vi "ValidateLumberjackConfigDTO.vi"(8 "error in (no error)":errorcluster, 11 "BaselineDTO":T1={"schemaVersion"="", "globalThreshold"="INFO", "defaultFileAppender"={"common"={"id"="", "threshold"="INFO", "filter"={"mode"="mirror", "levelMin"="INFO", "levelMax"="INFO", "tagPrefix"=""}, "queueBound"=0, "dropPolicy"="dropOldest", "useUTC"=FALSE}, "file"={"rootFolder"="", "maxFileSize"=0, "maxFileCount"=0, "baseName"="", "extension"="", "delimiter"="", "calendarFolderTree"=FALSE}}}) -> (0 "error out":errorcluster, 3 "MergedDTO":T1={"schemaVersion"="", "globalThreshold"="INFO", "defaultFileAppender"={"common"={"id"="", "threshold"="INFO", "filter"={"mode"="mirror", "levelMin"="INFO", "levelMax"="INFO", "tagPrefix"=""}, "queueBound"=0, "dropPolicy"="dropOldest", "useUTC"=FALSE}, "file"={"rootFolder"="", "maxFileSize"=0, "maxFileCount"=0, "baseName"="", "extension"="", "delimiter"="", "calendarFolderTree"=FALSE}}})   [LabVIEW 2026, in "Lumberjack.lvlib"]
doc: "Pure DTO validation. Fail-fast checks on a merged LumberjackConfigDTO, returning a descriptive error on the first invalid field: schema version, enum-name membership, file size, and filename safety of baseName and extension (SRS-LMBR-048, codes 5020-5039). Passes the DTO through on success. No I/O.\n\nMerged DTO -> descriptive error on first invalid field (else passthrough)."
uses:
  Lumberjack.lvlib
  <vilib>/Utility/Data Type/NI_Data Type.lvlib
  TypeDefs/ConfigDTO/FilterDTO.ctl
  TypeDefs/ConfigDTO/AppenderConfigDTO.ctl
  TypeDefs/ConfigDTO/FileAppenderConfigDTO.ctl
  TypeDefs/ConfigDTO/FileConfigDTO.ctl
  TypeDefs/ConfigDTO/LumberjackConfigDTO.ctl
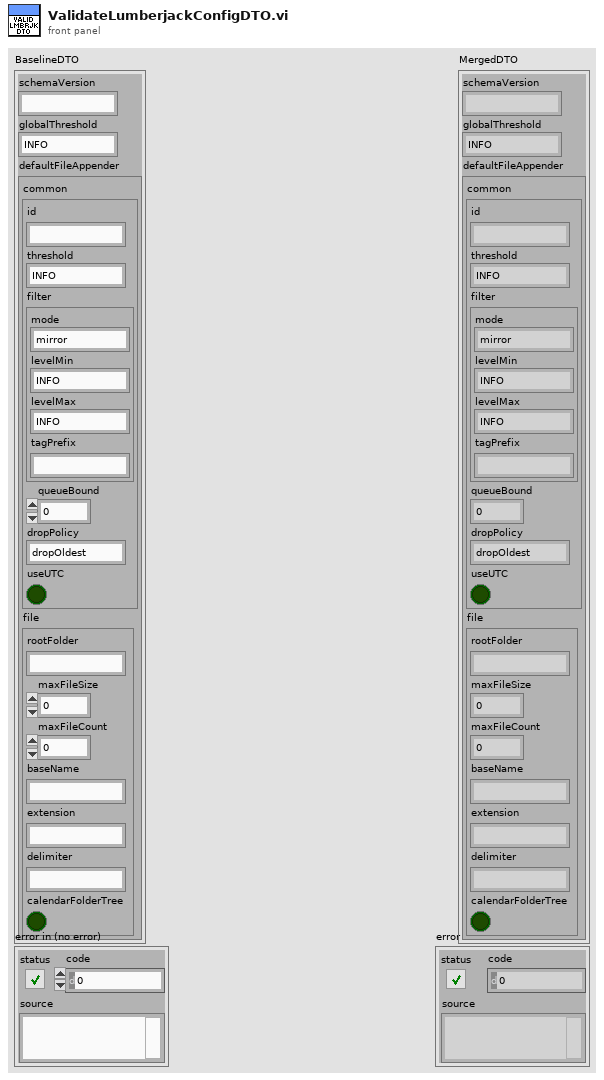
[diagram p1: front panel]
types:
  T1 = typedef "Lumberjack.lvlib/LumberjackConfigDTO.ctl" = cluster{"schemaVersion":string, "globalThreshold":string, "defaultFileAppender":T2}
  T2 = typedef "Lumberjack.lvlib/FileAppenderConfigDTO.ctl" = cluster{"common":T3, "file":T5}
  T3 = typedef "Lumberjack.lvlib/AppenderConfigDTO.ctl" = cluster{"id":string, "threshold":string, "filter":T4, "queueBound":i32, "dropPolicy":string, "useUTC":bool}
  T4 = typedef "Lumberjack.lvlib/FilterDTO.ctl" = cluster{"mode":string, "levelMin":string, "levelMax":string, "tagPrefix":string}
  T5 = typedef "Lumberjack.lvlib/FileConfigDTO.ctl" = cluster{"rootFolder":string, "maxFileSize":i64, "maxFileCount":i32, "baseName":string, "extension":string, "delimiter":string, "calendarFolderTree":bool}
  T6 = typedef "NI_Data Type.lvlib/Data Type.ctl" = enum8{"Invalid Type", "Void", "I8", "I16", "I32", "I64", "U8", "U16", "U32", "U64", "Single Float", "Double Float", "Extended Float", "Single Complex", "Double Complex", "Extended Complex", "Enum U8", "Enum U16", "Enum U32", "Enum U64", "Single Float With Unit", "Double Float With Unit", "Extended Float With Unit", "Single Complex with Unit", "Double Complex with Unit", "Extended Complex with Unit", "Boolean", "String", "Path", "Picture", "Tag", "Array", "Cluster", "Variant", "LV Variant", "Waveform", "Timestamp", "Digital Waveform", "Digital Data", "ExpressData", "Refnum", "External Data", "VI", "Poly VI", "LabVIEW Class Instance", "Fixed Point", "Set Collection", "Map Collection"}
  T7 = typedef "NI_Data Type.lvlib/Type Definition Info.ctl" = cluster{"Name":string, "Timestamp":u32}
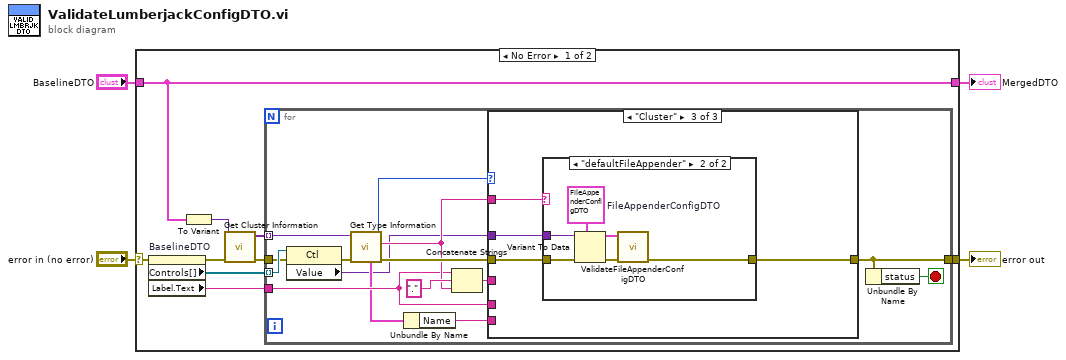
[diagram p0: block diagram]
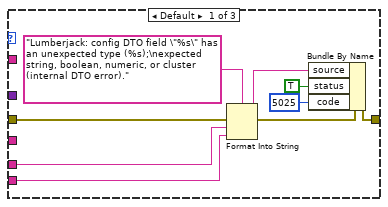
[diagram p2: hidden frame]
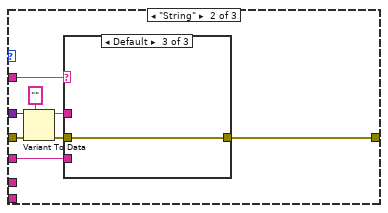
[diagram p3: hidden frame]
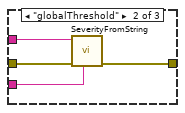
[diagram p5: hidden frame]
diagram:
  n1 = case shown="No Error" "error in (no error)" {
    selector: "error in (no error)" -> [w7 w63]
    tunnel: "BaselineDTO" -> [w5 w64]
    tunnel: [w5 w64] -> w2
    tunnel: [w6 w63] -> w1
    frame No Error {
      n2 = property on="BaselineDTO" class="Clust (strict)"(error in=w7) -> (error out=w11:errorcluster, "Controls[]"=w8:refnum<vi>[], "Label.Text"=w9:string)  [unwired: 1 in, 1 out]
      n3 = To Variant(anything=w5) -> (Variant=w10:variant)
      n4 = call <vilib>:"Get Cluster Information.vi"("error in (no error)"=w11, "variant"=w10) -> ("error out"=w12:errorcluster, "cluster elements"=w13:variant[])  [unwired: 8 in]
      n5 = for {
        tunnel: w13 -> [w23] mode=indexing
        tunnel: w12 -> [w16]
        tunnel: w9 -> [w22]
        tunnel: [w19] -> w6
        tunnel: w8 -> [w17] mode=indexing
        stop <- w18 stop-if-true
        n6 = property class="Ctl"(reference=w17, error in=w16) -> (error out=w14:errorcluster, "Value"=w15:variant)  [unwired: 1 out]
        n7 = call <vilib>:"Get Type Information.vi"("error in (no error)"=w14, "variant"=w23) -> ("error out"=w27:errorcluster, "name"=w24:string, "type"=w25:T6, "type definition info"=w21:T7)  [unwired: 5 in, 1 out]
        n8 = Unbundle By Name(w21) -> ("Name"=w20:string)
        n9 = Concatenate Strings(w22, "." ("string"), w24) -> (w26:string)
        n10 = case shown="\"Cluster\"" w25 {
          tunnel: w27 -> [w33 w43 w55]
          tunnel: w26 -> [_ w45 _]
          tunnel: w24 -> [_ w44 w53]
          tunnel: w15 -> [_ w41 w54]
          tunnel: w22 -> [w34 _ _]
          tunnel: [w30 w38 w52] -> w19
          tunnel: w20 -> [w31 _ _]
          frame Default {
            n11 = Format Into String(format string="Lumberjack: config DTO field \"%s\" has an unexpected type (%s);\nexpected string, boolean, numeric, or cluster (internal DTO error)." ("source"), error in=w33, w34, w31) -> (resulting string=w29:string, error out=w32:errorcluster)  [unwired: 1 in]
            n12 = Bundle By Name(cluster=w32, "source"=w29, "status"=TRUE, "code"=5025) -> (w30:errorcluster)
          }
          frame "String" {
            n13 = Variant To Data(error in=w43, type="", Variant=w41) -> (data=w39:string, error out=w42:errorcluster)
            n14 = case shown="Default" w44 {
              tunnel: w42 -> [w46 w50 w51]
              tunnel: w45 -> [_ w48 _]
              tunnel: w39 -> [_ w47 _]
              tunnel: [w46 w49 w51] -> w38
              frame "schemaVersion" {
              }
              frame "globalThreshold" {
                n15 = call "SeverityFromString.vi"("Context"=w48, "error in (no error)"=w50, "SeverityString"=w47) -> ("error out"=w49:errorcluster)  [unwired: 7 in, 1 out]
              }
              frame Default {
              }
            }
          }
          frame "Cluster" {
            n16 = case shown="\"defaultFileAppender\"" w53 {
              tunnel: w55 -> [w56 w62]
              tunnel: w54 -> [_ w61]
              tunnel: [w56 w58] -> w52
              frame Default {
              }
              frame "defaultFileAppender" {
                w57 = T2 {"common"={"id"="", "threshold"="INFO", "filter"={"mode"="Mirror", "levelMin"="INFO", "levelMax"="INFO", "tagPrefix"=""}, "queueBound"=0, "dropPolicy"="DropOldest", "useUTC"=FALSE}, "file"={"rootFolder"="", "maxFileSize"=0, "maxFileCount"=0, "baseName"="", "extension"="", "delimiter"="", "calendarFolderTree"=FALSE}}  # FileAppenderConfigDTO
                n17 = Variant To Data(error in=w62, type=w57, Variant=w61) -> (data=w59:T2, error out=w60:errorcluster)
                n18 = call "ValidateFileAppenderConfigDTO.vi"("error in (no error)"=w60, "FileAppenderConfigDTOin"=w59) -> ("error out"=w58:errorcluster)  [unwired: 8 in, 1 out]
              }
            }
          }
        }
        n19 = Unbundle By Name(w19) -> ("status"=w18:bool)
      }
    }
    frame Error {
    }
  }
  "error out" <- w1
  "MergedDTO" <- w2
